vi "Get Sheet By Name.vi"(8 "error in (no error)":errorcluster, 10 "Name":string, 11 "Excel Interface in":refnum<class "Excel Interface.lvclass">) -> (0 "error out":errorcluster, 1 "Sheet Found?":bool, 2 "Excel Sheet out":refnum<class "Excel Sheet.lvclass">, 3 "Excel Interface out":refnum<class "Excel Interface.lvclass">)   [LabVIEW 2016, in "Excel Interface.lvclass"]
uses:
  Excel Interface.lvclass
  Excel Sheet/Excel Sheet.lvclass
  Excel Interface.lvclass/Excel Interface.ctl
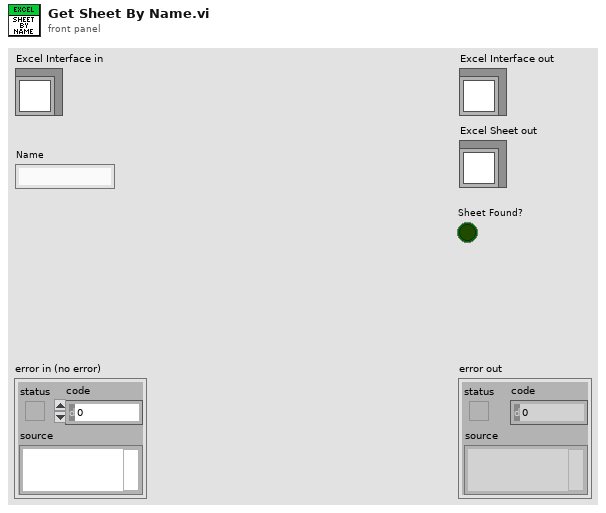
[diagram p1: front panel]
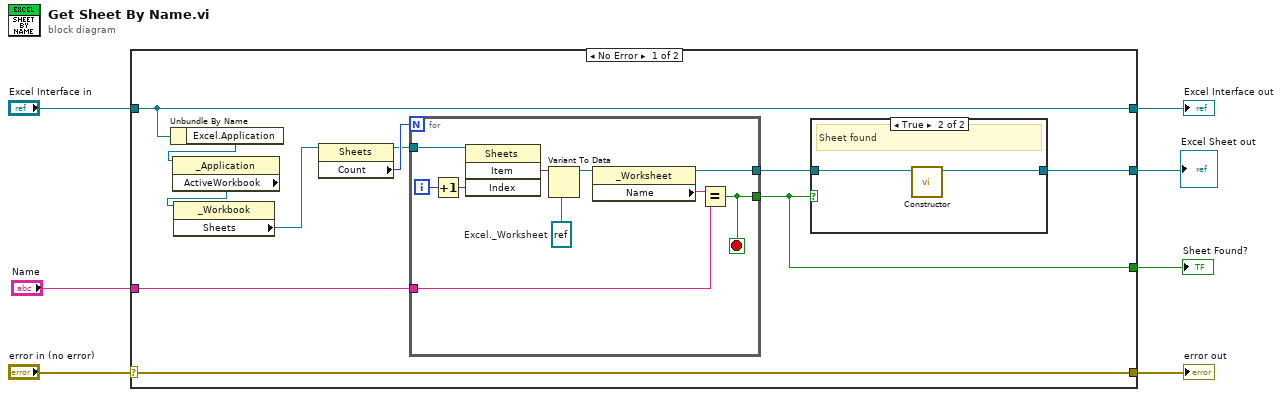
[diagram p0: block diagram]
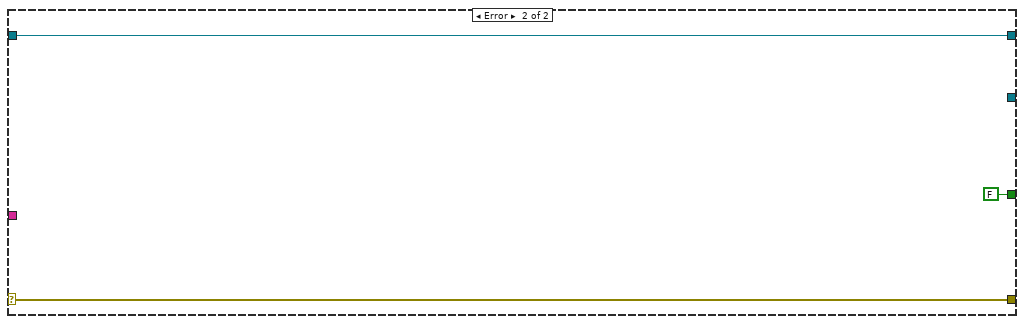
[diagram p3: hidden frame]
diagram:
  n1 = case shown="No Error" "error in (no error)" {
    selector: "error in (no error)" -> [w9 w33]
    tunnel: [w9 w33] -> w6
    tunnel: [w18 w32] -> w4
    tunnel: "Excel Interface in" -> [w18 w32]
    tunnel: "Name" -> [w12 _]
    tunnel: [w10 _] -> w2
    tunnel: [w8 FALSE] -> w1
    frame No Error {
      n2 = Unbundle By Name(w18) -> ("Excel.Application"=w17:refnum<k7>)
      n3 = property class="_Application"(reference=w17) -> ("ActiveWorkbook"=w16:refnum<k7>)  [unwired: 1 in, 2 out]
      n4 = property class="_Workbook"(reference=w16) -> ("Sheets"=w15:refnum<k7>)  [unwired: 1 in, 2 out]
      n5 = property class="Sheets"(reference=w15) -> (reference out=w13:refnum<k7>, "Count"=w14:i32)  [unwired: 1 in, 1 out]
      n6 = for {
        N: w14 -> [_]
        tunnel: w13 -> [w30]
        tunnel: w12 -> [w25]
        tunnel: [w24] -> w11
        tunnel: [w23] -> w8
        i -> [w22]
        stop <- w23 stop-if-true
        w29 = refnum<k7> refnum  # Excel._Worksheet
        n7 = Increment(x=w22) -> (x+1=w21:i32)
        n8 = invoke class="Sheets" method="Item"(reference=w30, "Index"=w21) -> ("Item"=w28:variant)  [unwired: 2 in, 3 out]
        n9 = Variant To Data(type=w29, Variant=w28) -> (data=w27:refnum<k7>)  [unwired: 1 in, 1 out]
        n10 = property class="_Worksheet"(reference=w27) -> (reference out=w24:refnum<k7>, "Name"=w26:string)  [unwired: 1 in, 1 out]
        n11 = Equal?(x=w26, y=w25) -> (x = y?=w23:bool)
      }
      n12 = case shown="True" w8 {
        tunnel: w11 -> [_ w20]
        tunnel: [_ w19] -> w10
        frame False {
          # "Sheet not found"
        }
        frame True {
          # "Sheet found"
          n13 = call "Constructor.vi"("Worksheet"=w20) -> ("Excel Sheet out"=w19:refnum<class "Excel Sheet.lvclass">)  [unwired: 10 in]
        }
      }
    }
    frame Error {
    }
  }
  "error out" <- w6
  "Excel Interface out" <- w4
  "Excel Sheet out" <- w2
  "Sheet Found?" <- w1
